vi "GDSString_FindWord.vi"(0 "Text":string, 1 "StringStartOffset(Default=-1 => 0 for Forward, StrLenght for Backwards)":i32=-1, 2 "PatternMatchingDelimiter(\\s\\t\\r\\n)":string="\\s\\t\\r\\n", 3 "Search Backwards":bool, 4 "AllowedWords(PatternMatching)":string[](array[string]), 5 "error in (no error)":errorcluster, 6 "GetNext-X_Words(1,-1=All)":i32=1) -> (14 "NextWord":string, 15 "IndexAfterMatch(Or before when searching Backwards)":i32=1, 16 "NextWords":string[](array[string]), 17 "IndexAfterMatches(Or before when searching Backwards)":i32[](array[numeric]), 18 "IndexAfterLastMatch":i32=1, 19 "error out":errorcluster)   [LabVIEW 2012]
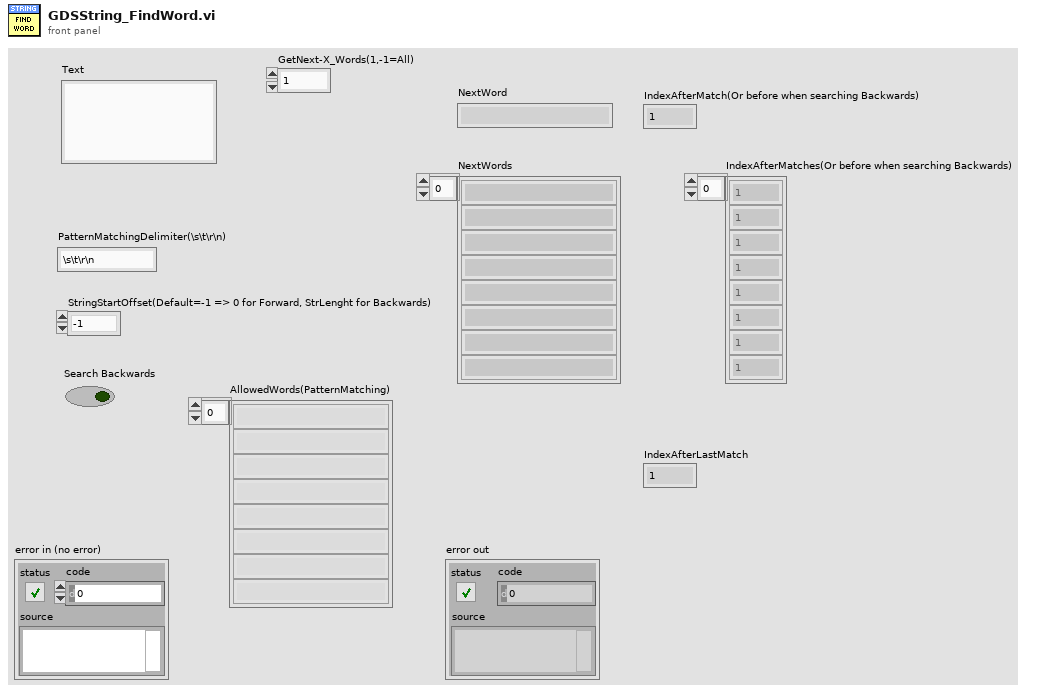
[diagram p1: front panel]
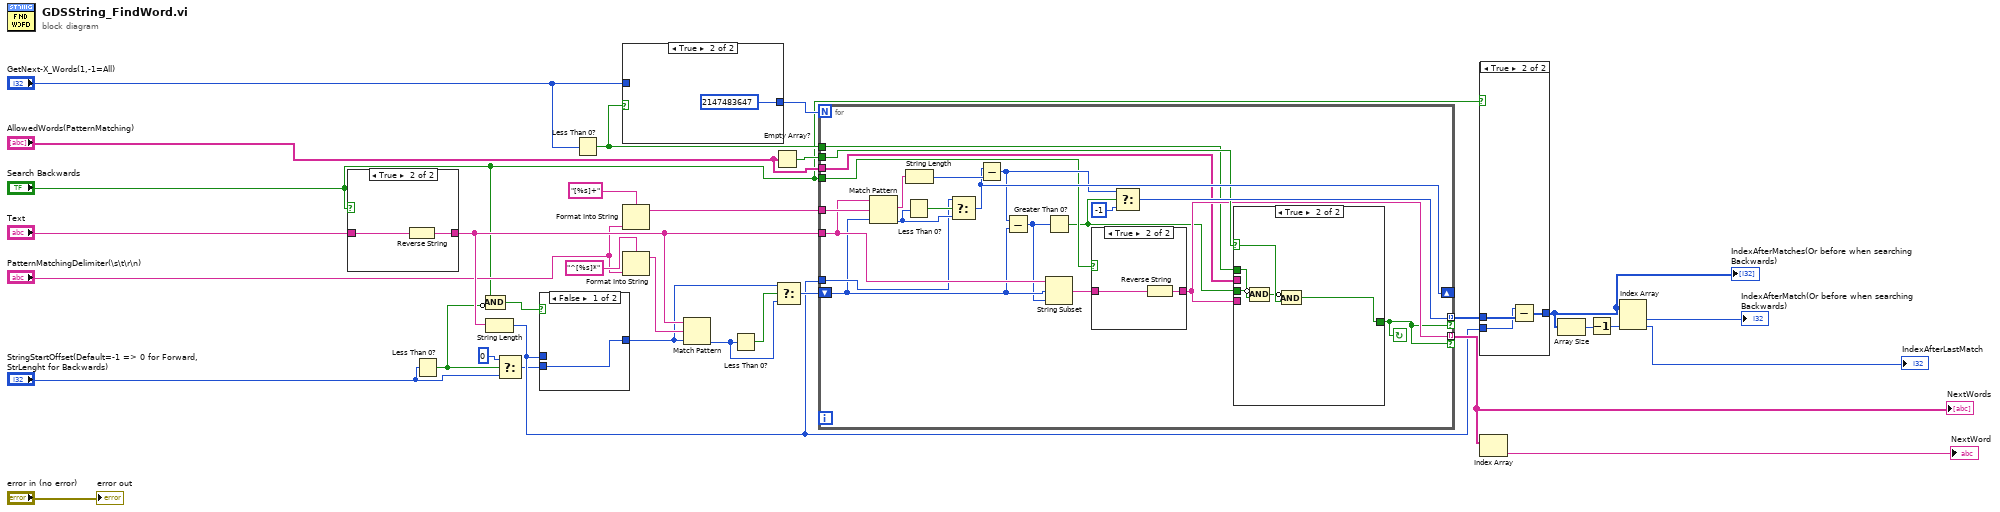
[diagram p0: block diagram]
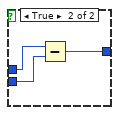
[diagram p2: hidden frame]
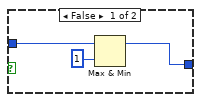
[diagram p3: hidden frame]
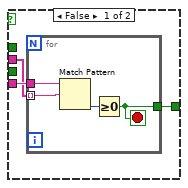
[diagram p4: hidden frame]
diagram:
  n1 = case shown="True" "Search Backwards" {
    tunnel: "Text" -> [w33 w35]
    tunnel: [w33 w34] -> w25
    frame False {
    }
    frame True {
      n2 = Reverse String(1:w35) -> (0:w34:string)
    }
  }
  n3 = Less Than 0?(x="StringStartOffset(Default=-1 => 0 for Forward, StrLenght for Backwards)") -> (x < 0?=w3:bool)
  n4 = Compound Arithmetic op=AND("Search Backwards", invert w3) -> (w1:bool)
  n5 = String Length(string=w25) -> (length=w6:i32)
  n6 = Select(t=0, s=w3, f="StringStartOffset(Default=-1 => 0 for Forward, StrLenght for Backwards)") -> (s? t:f=w5:i32)
  n7 = case shown="False" w1 {
    tunnel: w5 -> [w36 w38]
    tunnel: [w36 w37] -> w4
    tunnel: w6 -> [_ w39]
    frame False {
    }
    frame True {
      n8 = Subtract(x=w39, y=w38) -> (x-y=w37:i32)
    }
  }
  n9 = Less Than 0?(x="GetNext-X_Words(1,-1=All)") -> (x < 0?=w12:bool)
  n10 = case shown="True" w12 {
    tunnel: [w41 2147483647] -> w26
    tunnel: "GetNext-X_Words(1,-1=All)" -> [w40 _]
    frame False {
      n11 = Max & Min(x=w40, y=1) -> (max(x,y)=w41:i32)  [unwired: 1 out]
    }
    frame True {
    }
  }
  n12 = Format Into String(format string="[%s]+", "PatternMatchingDelimiter(\\s\\t\\r\\n)") -> (resulting string=w29:string)  [unwired: 2 in, 1 out]
  n13 = Format Into String(format string="^[%s]*", "PatternMatchingDelimiter(\\s\\t\\r\\n)") -> (resulting string=w21:string)  [unwired: 2 in, 1 out]
  n14 = Match Pattern(string=w25, regular expression=w21, offset (0)=w4) -> (offset past match=w18:i32)  [unwired: 3 out]
  n15 = Less Than 0?(x=w18) -> (x < 0?=w19:bool)
  n16 = Empty Array?(array="AllowedWords(PatternMatching)") -> (empty?=w15:bool)
  n17 = Select(t=w4, s=w19, f=w18) -> (s? t:f=w7:i32)
  n18 = for {
    N: w26 -> [_]
    tunnel: w25 -> [w61]
    tunnel: w29 -> [w64]
    tunnel: [w52] -> w20 mode=indexing if=w46
    shift-right: [w56] -> _
    shift-left: w7 -> [w57]
    tunnel: w6 -> [w58]
    tunnel: [w48] -> w16 mode=indexing if=w46
    tunnel: "Search Backwards" -> [w51]
    tunnel: w15 -> [w49]
    tunnel: "AllowedWords(PatternMatching)" -> [w47]
    tunnel: w12 -> [w44]
    stop <- w46 continue-if-true
    n19 = Match Pattern(string=w61, regular expression=w64, offset (0)=w57) -> (match substring=w63:string, offset past match=w59:i32)  [unwired: 2 out]
    n20 = Less Than 0?(x=w59) -> (x < 0?=w60:bool)
    n21 = String Length(string=w63) -> (length=w62:i32)
    n22 = Select(t=w58, s=w60, f=w59) -> (s? t:f=w56:i32)
    n23 = Subtract(x=w56, y=w62) -> (x-y=w54:i32)
    n24 = Subtract(x=w54, y=w57) -> (x-y=w55:i32)
    n25 = Greater Than 0?(x=w55) -> (x > 0?=w45:bool)
    n26 = String Subset(string=w61, offset (0)=w57, length (rest)=w55) -> (substring=w50:string)
    n27 = case shown="True" w51 {
      tunnel: w50 -> [w77 w79]
      tunnel: [w77 w78] -> w48
      frame False {
      }
      frame True {
        n28 = Reverse String(1:w79) -> (0:w78:string)
      }
    }
    n29 = Select(t=w54, s=w45, f=-1) -> (s? t:f=w52:i32)
    n30 = case shown="True" w49 {
      selector: w49 -> [_ w76]
      tunnel: [w65 w75] -> w46
      tunnel: w48 -> [w67 _]
      tunnel: w47 -> [w66 _]
      tunnel: w45 -> [_ w74]
      tunnel: w44 -> [_ w73]
      frame False {
        n31 = for {
          tunnel: w67 -> [w71]
          tunnel: w66 -> [w70] mode=indexing
          tunnel: [w68] -> w65
          stop <- w68 stop-if-true
          n32 = Match Pattern(string=w71, regular expression=w70) -> (offset past match=w69:i32)  [unwired: 1 in, 3 out]
          n33 = Greater Or Equal To 0?(x=w69) -> (x >= 0?=w68:bool)
        }
      }
      frame True {
        n34 = Compound Arithmetic op=AND(invert w74, w73) -> (w72:bool)
        n35 = Compound Arithmetic op=AND(invert w72, w76) -> (w75:bool)
      }
    }
  }
  "NextWords" <- w16
  n36 = case shown="True" "Search Backwards" {
    tunnel: w20 -> [w80 w83]
    tunnel: [w80 w81] -> w11
    tunnel: w6 -> [_ w82]
    frame False {
    }
    frame True {
      n37 = Subtract(x=w82, y=w83) -> (x-y=w81:i32[])
    }
  }
  "IndexAfterMatches(Or before when searching Backwards)" <- w11
  n38 = Index Array(array=w16) -> (element=→"NextWord":string)  [unwired: 1 in]
  n39 = Array Size(array=w11) -> (size(s)=w10:i32)
  n40 = Decrement(x=w10) -> (x-1=w9:i32)
  n41 = Index Array(array=w11, index #2=w9) -> (element #1=→"IndexAfterMatch(Or before when searching Backwards)":i32, element #2=→"IndexAfterLastMatch":i32)  [unwired: 1 in]
  "error out" <- "error in (no error)"
